vi "Pool Queue ASCII Correction.vi"(11 "Uncorrected Data":string) -> (3 "Corrected Data":string)   [LabVIEW 2012]
doc: "This VI scans the input string for the ASCII character string (located within parentheses). Once found, it removes all commas from the string."
panel:
  out "Loop Count":i32
  out "Loop2":i32
  out "Loop 1":i32
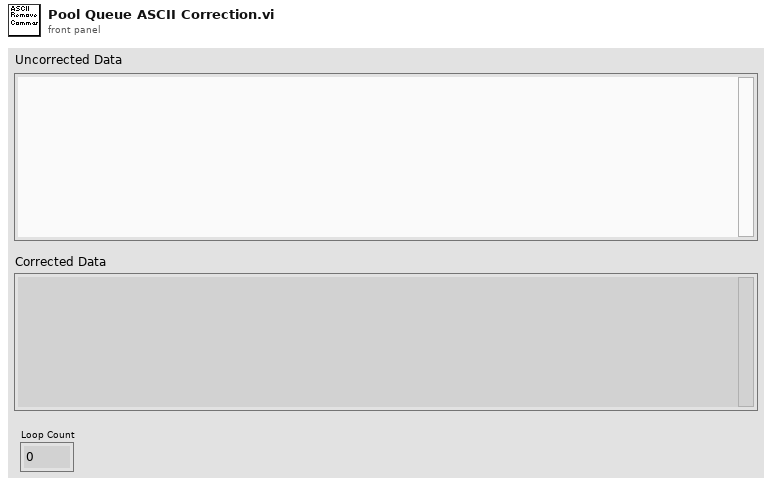
[diagram p1: front panel]
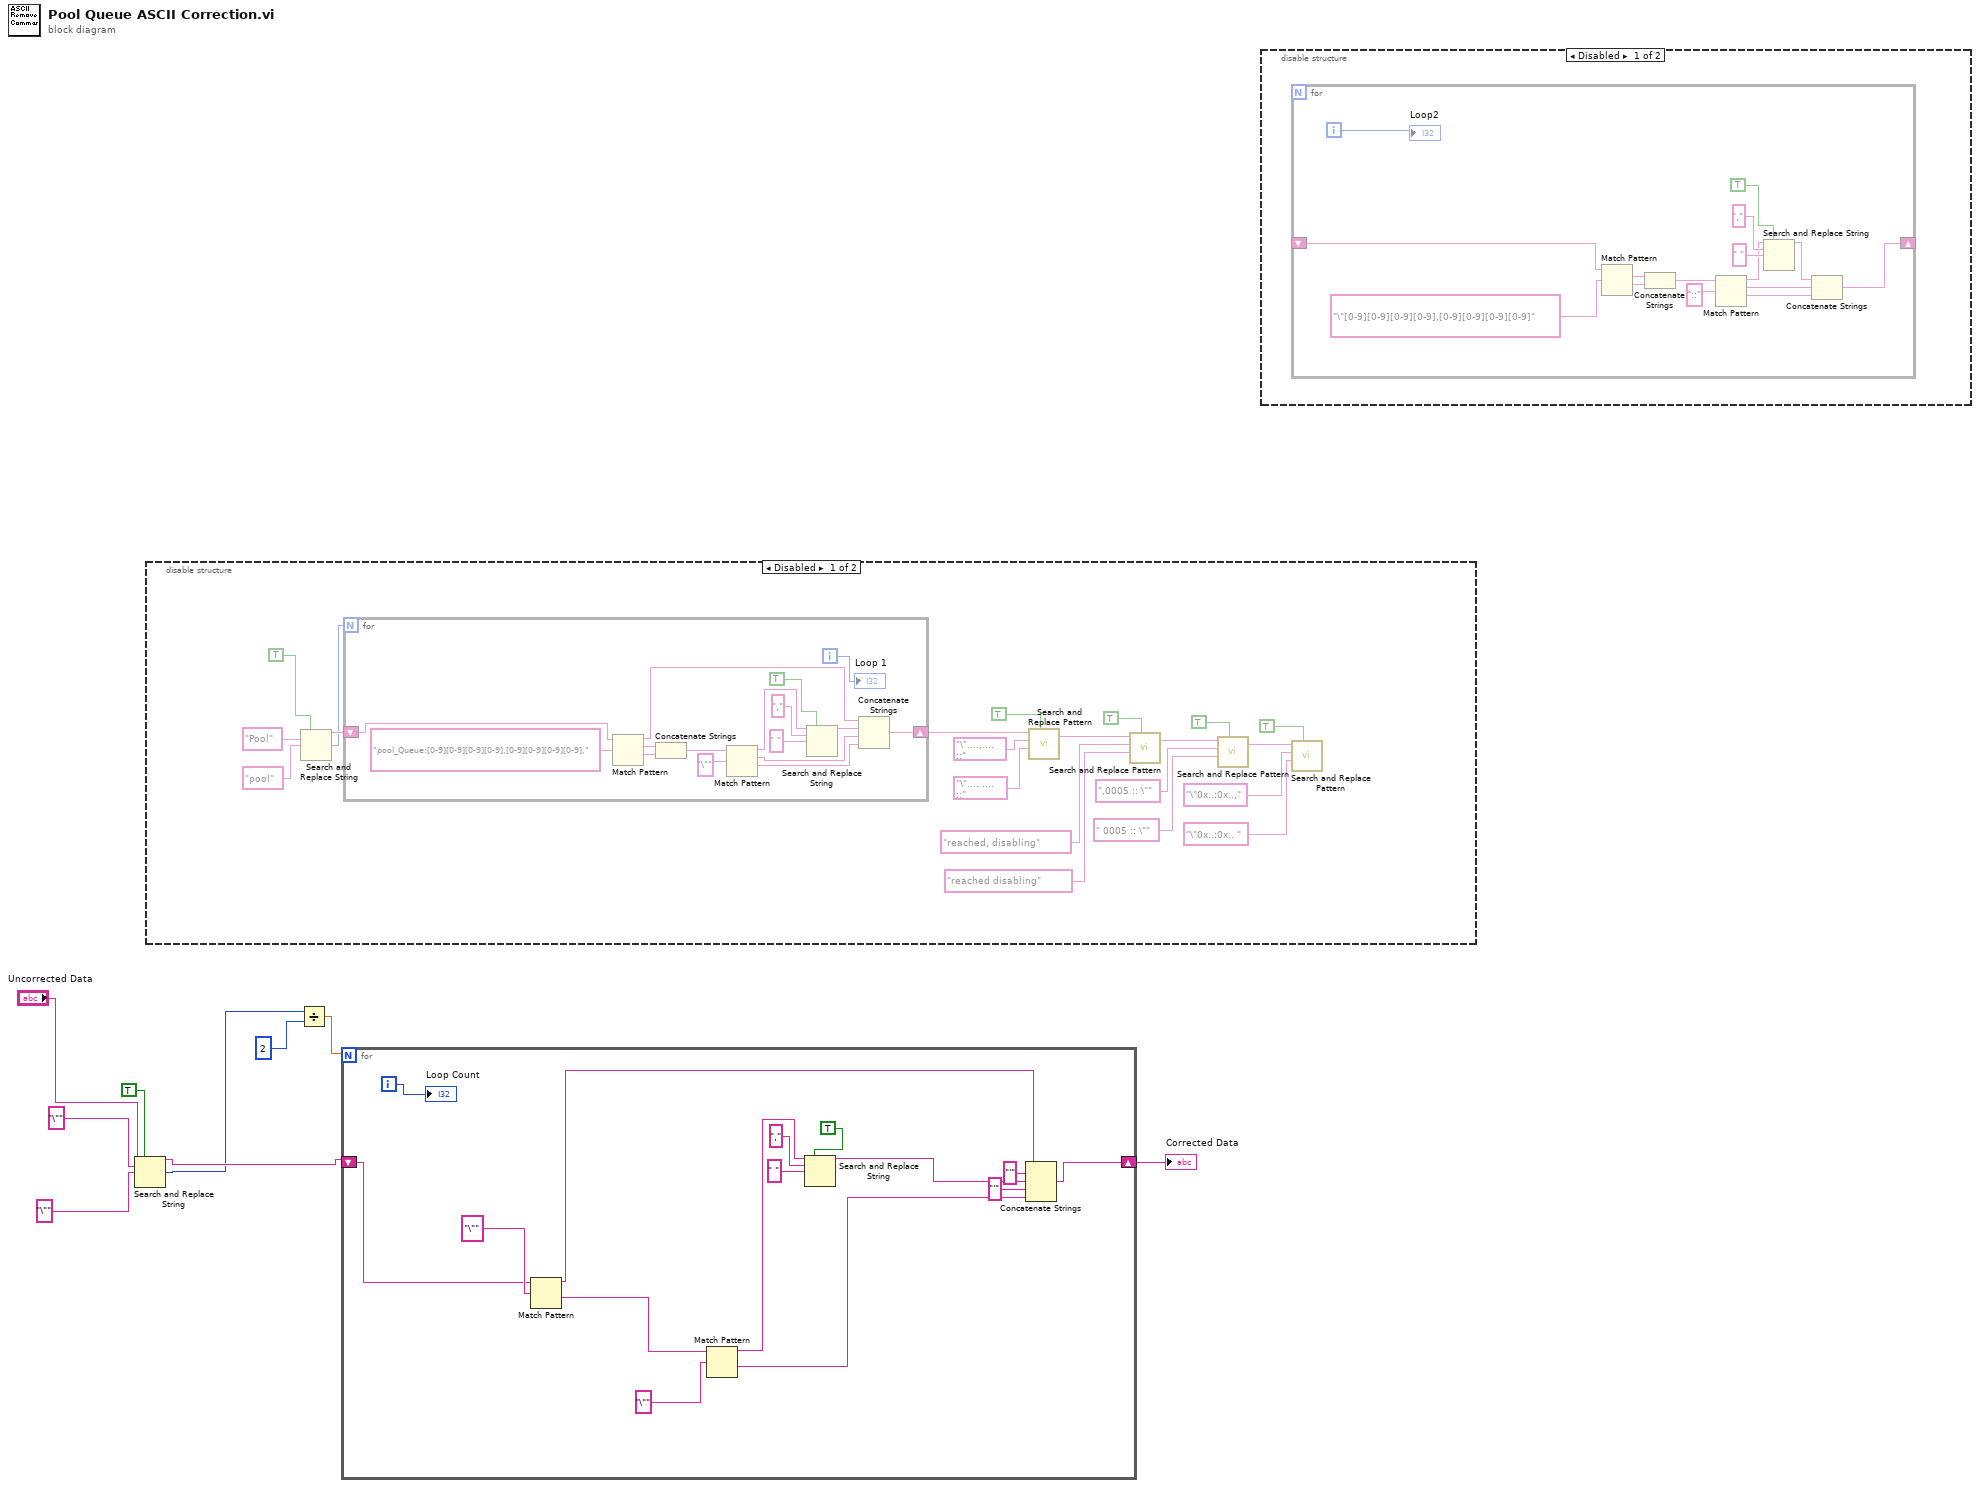
[diagram p0: block diagram]
diagram:
  n1 = Search and Replace String(replace all?=TRUE ("replace all? (F)"), input string="Uncorrected Data", search string="\"", replace string="\"" ("replace string (\"\")")) -> (result string=w8:string, number of replacements=w7:i32)  [unwired: 4 in, 2 out]
  n2 = disable-structure shown="Disabled" {
    frame Disabled {
      n3 = Search and Replace String(replace all?=TRUE ("replace all? (F)"), search string="Pool", replace string="pool" ("replace string (\"\")")) -> (result string=w24:string, number of replacements=w23:i32)  [unwired: 5 in, 2 out]
      n4 = for {
        N: w23 -> [_]
        shift-right: [w36] -> w16
        shift-left: w24 -> [w37]
        i -> [w45]
        n5 = Match Pattern(string=w37, regular expression="pool_Queue:[0-9][0-9][0-9][0-9],[0-9][0-9][0-9][0-9]," ("search string")) -> (before substring=w39:string, match substring=w44:string, after substring=w43:string)  [unwired: 1 in, 1 out]
        n6 = Concatenate Strings(w44, w43) -> (w42:string)
        n7 = Match Pattern(string=w42, regular expression="\"") -> (before substring=w40:string, match substring=w31:string, after substring=w32:string)  [unwired: 1 in, 1 out]
        n8 = Search and Replace String(replace all?=TRUE ("replace all? (F)"), input string=w40, search string=",", replace string=" " ("replace string (\"\")")) -> (result string=w38:string)  [unwired: 4 in, 3 out]
        n9 = Concatenate Strings(w39, w38, w31, w32) -> (w36:string)
        "Loop 1" <- w45
      }
      n10 = call <vilib>:"Search and Replace Pattern.vi"("string"=w16, "regular expression (\"\")"="\"....,.... ::" ("search string"), "replace string (\"\")"="\".... .... ::" ("replace string (\"\")"), "replace all? (F)"=TRUE) -> ("result string"=w15:string)  [unwired: 1 in, 1 out]
      n11 = call <vilib>:"Search and Replace Pattern.vi"("string"=w15, "regular expression (\"\")"="reached, disabling" ("search string"), "replace string (\"\")"="reached disabling" ("replace string (\"\")"), "replace all? (F)"=TRUE) -> ("result string"=w14:string)  [unwired: 1 in, 1 out]
      n12 = call <vilib>:"Search and Replace Pattern.vi"("string"=w14, "regular expression (\"\")"=",0005 :: \"" ("regular expression (\"\")"), "replace string (\"\")"=" 0005 :: \"" ("replace string (\"\")"), "replace all? (F)"=TRUE) -> ("result string"=w12:string)  [unwired: 1 in, 1 out]
      n13 = call <vilib>:"Search and Replace Pattern.vi"("string"=w12, "regular expression (\"\")"="\"0x..:0x..," ("replace string (\"\")"), "replace string (\"\")"="\"0x..:0x.. " ("regular expression (\"\")"), "replace all? (F)"=TRUE) -> ()  [unwired: 1 in, 2 out]
    }
    frame Enabled {
    }
  }
  n14 = Divide(x=w7, y=2) -> (x/y=w5:dbl)
  n15 = for {
    N: w5 -> [_]
    shift-right: [w55] -> w4
    shift-left: w8 -> [w56]
    i -> [w60]
    n16 = Match Pattern(string=w56, regular expression="\"" ("search string")) -> (before substring=w49:string, after substring=w50:string)  [unwired: 1 in, 2 out]
    n17 = Match Pattern(string=w50, regular expression="\"") -> (before substring=w58:string, after substring=w51:string)  [unwired: 1 in, 2 out]
    n18 = Search and Replace String(replace all?=TRUE ("replace all? (F)"), input string=w58, search string=",", replace string=" " ("replace string (\"\")")) -> (result string=w57:string)  [unwired: 4 in, 3 out]
    n19 = Concatenate Strings(w49, "'" ("string"), w57, "'" ("string"), w51) -> (w55:string)
    "Loop Count" <- w60
  }
  "Corrected Data" <- w4
  n20 = disable-structure shown="Disabled" {
    frame Disabled {
      n21 = for {
        shift-right: [w62] -> _
        shift-left: _ -> [w64]
        i -> [w63]
        n22 = Match Pattern(string=w64, regular expression="\"[0-9][0-9][0-9][0-9],[0-9][0-9][0-9][0-9]" ("search string")) -> (match substring=w66:string, after substring=w67:string)  [unwired: 1 in, 2 out]
        n23 = Concatenate Strings(w66, w67) -> (w68:string)
        n24 = Match Pattern(string=w68, regular expression="::") -> (before substring=w70:string, match substring=w76:string, after substring=w75:string)  [unwired: 1 in, 1 out]
        n25 = Search and Replace String(replace all?=TRUE ("replace all? (F)"), input string=w70, search string=",", replace string=" " ("replace string (\"\")")) -> (result string=w71:string)  [unwired: 4 in, 3 out]
        n26 = Concatenate Strings(w71, w76, w75) -> (w62:string)
        "Loop2" <- w63
      }
    }
    frame Enabled {
    }
  }
